vi "Add Subscription.vi"(8 "error in (no error)":errorcluster, 9 "SessionMailbox":refnum<queue>, 10 "Topic Subscription":T1, 11 "MQTT Server":refnum<class "Server.lvclass">) -> (0 "error out":errorcluster, 1 "Failed":bool, 3 "MQTT Server":refnum<class "Server.lvclass">)   [LabVIEW 2013, in "MQTT Server.lvlib" / "Server.lvclass"]
uses:
  Server.lvclass
  <vilib>/LabVIEW Open Source Project/MQTT Control Packets/Control Packets/SUBSCRIBE/Topic Subscription -- cluster.ctl
  <vilib>/LabVIEW Open Source Project/MQTT Control Packets/Control Packets/ControlPacket/QualityOfService -- enum.ctl
  <vilib>/LabVIEW Open Source Project/MQTT Connection/MQTT_Base/Base Class/Response -- cluster.ctl
  <vilib>/LabVIEW Open Source Project/MQTT Control Packets/Control Packets/ControlPacket/ControlPacket.lvclass
  Server.lvclass/Server.ctl
  Subscription/_Subscription.lvclass/_Subscription.ctl
  TopicFilter/_TopicFilter.lvclass/_TopicFilter.ctl
  Subscription/_Subscription.lvclass
  StoredSessions/StoredSessions.lvclass
  <vilib>/LabVIEW Open Source Project/MQTT Connection/MQTT_Base/Base Class/MQTT_Base.lvclass
  <vilib>/LabVIEW Open Source Project/MQTT Control Packets/Control Packets/SUBSCRIBE/SUBSCRIBE.lvclass
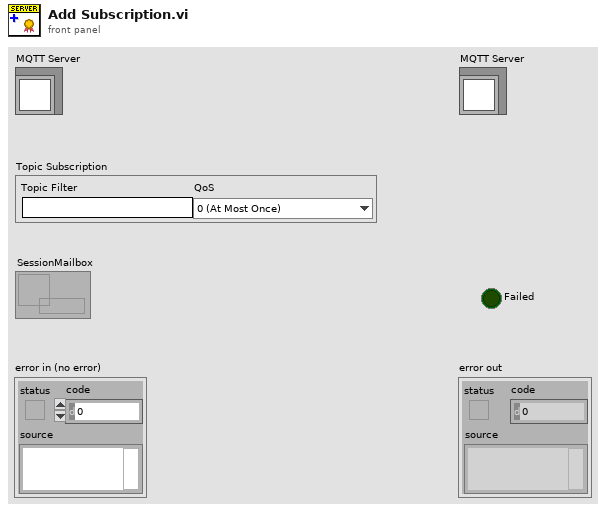
[diagram p1: front panel]
types:
  T1 = typedef "MQTT_Control_Packets.lvlib/SUBSCRIBE.lvclass/Topic Subscription -- cluster.ctl" = cluster{"Topic Filter":string, "QoS":T2}
  T2 = typedef "MQTT_Control_Packets.lvlib/ControlPacket.lvclass/QualityOfService -- enum.ctl" = enum16{"0 (At Most Once)", "1 (At Least Once)", "2 (Exactly Once)"}
  T3 = typedef "MQTT Server.lvlib/Server.lvclass/Private Events -- cluster.ctl" = cluster{"Inbound Packet":refnum<user-event>, "Inbound Ack":refnum<user-event>}
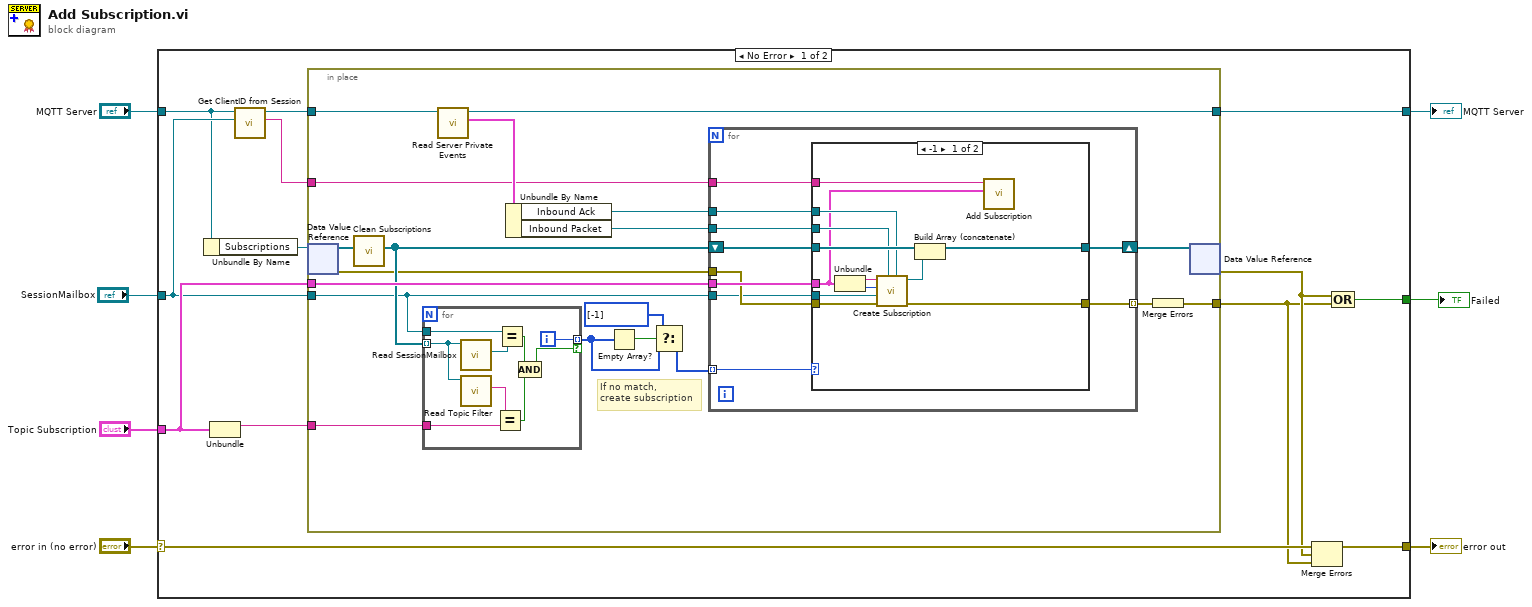
[diagram p0: block diagram]
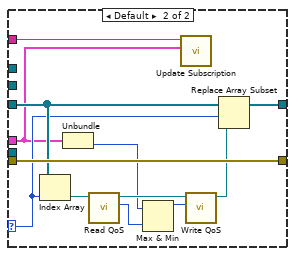
[diagram p2: hidden frame]
diagram:
  n1 = case shown="No Error" "error in (no error)" {
    selector: "error in (no error)" -> [w19 w84]
    tunnel: [w18 w84] -> w6
    tunnel: [w12 w83] -> w4
    tunnel: "MQTT Server" -> [w10 w83]
    tunnel: "Topic Subscription" -> [w16 _]
    tunnel: [w13 _] -> w2
    tunnel: "SessionMailbox" -> [w11 _]
    frame No Error {
      n2 = Unbundle By Name(w10) -> ("Subscriptions"=w20:refnum<data-value>)
      n3 = Unbundle(w16) -> ("Topic Filter"=w17:string)  [unwired: 1 out]
      n4 = call "Get ClientID from Session.vi"("SessionMailbox"=w11, "MQTT Server"=w10) -> ("Client ID"=w8:string, "MQTT Server"=w9:refnum<class "Server.lvclass">)  [unwired: 6 in, 2 out]
      n5 = in-place {
        in-place-border: w17 -> [w32]
        in-place-border: w9 -> [w25]
        in-place-border: w11 -> [w33]
        in-place-border: w16 -> [w38]
        in-place-border: [w31] -> w14
        in-place-border: [w21] -> w12
        in-place-border: w8 -> [w22]
        # "If no match,\ncreate subscription"
        n6 = in-place-dvr #1(w20) -> (w36:refnum<class "_Subscription.lvclass">[], w34:errorcluster)
        n7 = call "Clean Subscriptions.vi"("Subscriptions in"=w36) -> ("Subscriptions"=w35:refnum<class "_Subscription.lvclass">[])  [unwired: 10 in]
        n8 = for {
          tunnel: w35 -> [w82] mode=indexing
          tunnel: w33 -> [w80]
          tunnel: w32 -> [w78]
          tunnel: [w75] -> w28 mode=indexing if=w74
          i -> [w75]
          n9 = call "Read SessionMailbox.vi"("Subscription in"=w82) -> ("SessionMailbox"=w81:refnum<queue>)  [unwired: 8 in, 2 out]
          n10 = call "Read Topic Filter.vi"("Subscription in"=w82) -> ("Topic Filter"=w79:string)  [unwired: 7 in, 3 out]
          n11 = Equal?(x=w79, y=w78) -> (x = y?=w76:bool)
          n12 = Equal?(x=w80, y=w81) -> (x = y?=w77:bool)
          n13 = Compound Arithmetic op=AND(w77, w76) -> (w74:bool)
        }
        n14 = call "Read Server Private Events.vi"("Server in"=w25) -> ("Server Private Events"=w26:T3, "Server out"=w21:refnum<class "Server.lvclass">)  [unwired: 8 in, 1 out]
        n15 = Unbundle By Name(w26) -> ("Inbound Ack"=w23:refnum<user-event>, "Inbound Packet"=w24:refnum<user-event>)
        n16 = Empty Array?(array=w28) -> (empty?=w30:bool)
        n17 = Select(t=i32[] [-1], s=w30, f=w28) -> (s? t:f=w29:i32[])
        n18 = for {
          tunnel: w38 -> [w48]
          tunnel: [w47] -> w37 mode=indexing
          tunnel: w34 -> [w45]
          tunnel: w33 -> [w44]
          shift-right: [w49] -> w39
          shift-left: w35 -> [w46]
          tunnel: w29 -> [w43] mode=indexing
          tunnel: w24 -> [w42]
          tunnel: w23 -> [w41]
          tunnel: w22 -> [w40]
          n19 = case shown="-1" w43 {
            selector: w43 -> [_ w70]
            tunnel: [w61 w73] -> w49
            tunnel: w46 -> [w60 w71]
            tunnel: w44 -> [w59 _]
            tunnel: w48 -> [w50 w62]
            tunnel: [w56 w72] -> w47
            tunnel: w45 -> [w55 w72]
            tunnel: w42 -> [w54 _]
            tunnel: w41 -> [w53 _]
            tunnel: w40 -> [w51 w63]
            frame -1 {
              n20 = Unbundle(w50) -> ("Topic Filter"=w58:string, "QoS"=w57:T2)
              n21 = call "Create Subscription.vi"("Inbound Ack"=w53, "Inbound Message"=w54, "error in (no error)"=w55, "SessionMailbox"=w59, "QoS"=w57, "Topic Filter"=w58) -> ("error out"=w56:errorcluster, "Subscription out"=w52:refnum<class "_Subscription.lvclass">)  [unwired: 4 in]
              n22 = Build Array (concatenate)(w60, w52) -> (w61:refnum<class "_Subscription.lvclass">[])
              n23 = call "Add Subscription.vi"("Topic Subscription"=w50, "Client ID"=w51) -> ()  [unwired: 9 in, 1 out]
            }
            frame Default {
              n24 = Index Array(array=w71, index=w70) -> (element=w64:refnum<class "_Subscription.lvclass">)
              n25 = Unbundle(w62) -> ("QoS"=w67:T2)  [unwired: 1 out]
              n26 = call "Read QoS.vi"("Subscription in"=w64) -> ("QoS"=w68:T2, "Subscription out"=w69:refnum<class "_Subscription.lvclass">)  [unwired: 8 in, 1 out]
              n27 = Max & Min(x=w67, y=w68) -> (max(x,y)=w66:u16)  [unwired: 1 out]
              n28 = call "Update Subscription.vi"("Topic Subscription"=w62, "Client ID"=w63) -> ()  [unwired: 9 in, 1 out]
              n29 = call "Write QoS.vi"("QoS"=w66, "Subscription in"=w69) -> ("Subscription out"=w65:refnum<class "_Subscription.lvclass">)  [unwired: 8 in, 1 out]
              n30 = Replace Array Subset(array=w71, new element=w65, index=w70) -> (w73:refnum<class "_Subscription.lvclass">[])
            }
          }
        }
        n31 = Merge Errors(w37) -> (w31:errorcluster)
        n32 = in-place-dvr #1(w39) -> (w15:errorcluster)  [unwired: 1 out]
      }
      n33 = Merge Errors(w19, w15, w14) -> (w18:errorcluster)
      n34 = Compound Arithmetic op=OR(w15, w14) -> (w13:bool)
    }
    frame Error {
    }
  }
  "error out" <- w6
  "MQTT Server" <- w4
  "Failed" <- w2
